vi "Main.vi"() -> ()   [LabVIEW 2018]
doc: "The myRIO Project template acquires acceleration data from the onboard accelerometer and displays the changes of acceleration values in a waveform chart."
uses:
  <vilib>/myRIO/Instrument Drivers/Onboard IO/SPI/typedefs/SPI User Configuration.ctl
  <vilib>/myRIO/Common/Instrument Driver Framework/myRIO v1.0/SPI/typedefs/SPI Clock Phase.ctl
  <vilib>/myRIO/Common/Instrument Driver Framework/myRIO v1.0/SPI/typedefs/SPI Clock Polarity.ctl
  <vilib>/myRIO/Common/Instrument Driver Framework/myRIO v1.0/SPI/typedefs/SPI Data Direction.ctl
  <vilib>/myRIO/Common/Instrument Driver Framework/myRIO v1.0/SPI/typedefs/SPI Frame Length.ctl
  <vilib>/myRIO/Common/Instrument Driver Framework/myRIO v1.0/UART/vis/myRIO v1.0 Close UART.vi
  <vilib>/myRIO/Common/Instrument Driver Framework/Utilities/vis/FPGA Ref Manager.vi
  <vilib>/myRIO/Common/Instrument Driver Framework/myRIO v1.0/myRIO v1.0 Reset FPGA.vi
  <vilib>/myRIO/Common/Instrument Driver Framework/myRIO v1.0/IRQ/vis/myRIO v1.0 IRQ Info FGV.vi
  <vilib>/myRIO/Common/Instrument Driver Framework/myRIO v1.0/IRQ/vis/myRIO v1.0 Timer IRQ Info FGV.vi
  <vilib>/myRIO/Common/Instrument Driver Framework/myRIO v1.0/IRQ/vis/myRIO v1.0 ISR Agent.vi
  <vilib>/myRIO/Instrument Drivers/Utilities/Utilities.lvlib
  <vilib>/myRIO/Instrument Drivers/Onboard IO/SPI/SPI.lvlib
panel:
  out "Data Channel 0":u16[](array[numeric])
  out "Ch0 Distance (cm)":dbl
  out "Ch1 Distance (cm)":dbl
  out "Ch2 Distance (cm)":dbl
  out "Readings good?":bool[](array[boolean])
  out "error out":errorcluster
  in  "Stop":bool
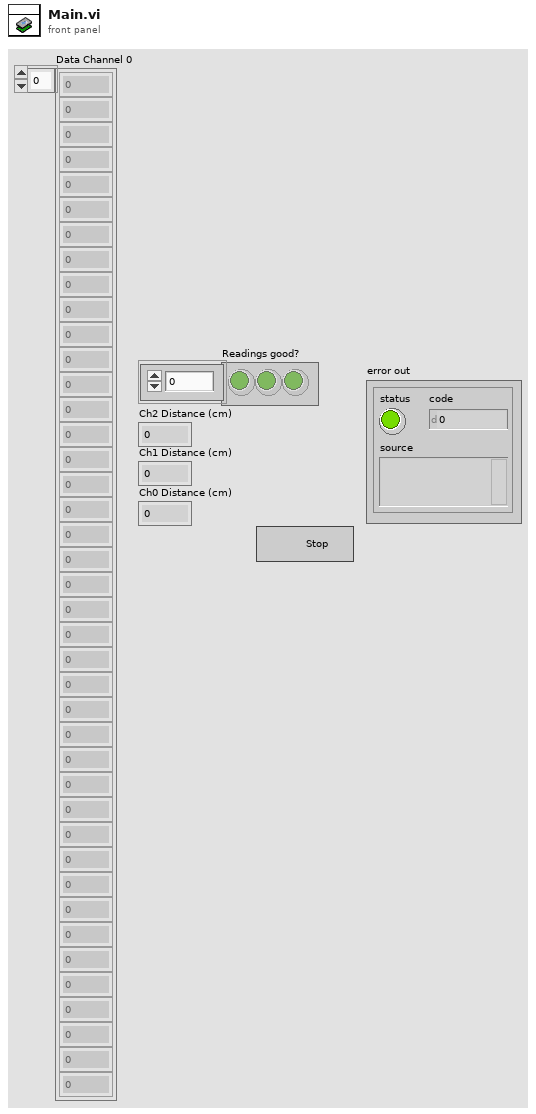
[diagram p1: front panel]
types:
  T1 = typedef "SPI.lvlib/SPI User Configuration.ctl" = cluster{"Frequency [Hz]":dbl, "Clock Phase":T2, "Clock Polarity":T3, "Data Direction":T4, "Frame Length":T5}
  T2 = typedef "SPI Clock Phase.ctl" = enum8{"Leading", "Trailing"}
  T3 = typedef "SPI Clock Polarity.ctl" = enum8{"Low", "High"}
  T4 = typedef "SPI Data Direction.ctl" = enum8{"Most significant bit first", "Least significant bit first"}
  T5 = typedef "SPI Frame Length.ctl" = u8
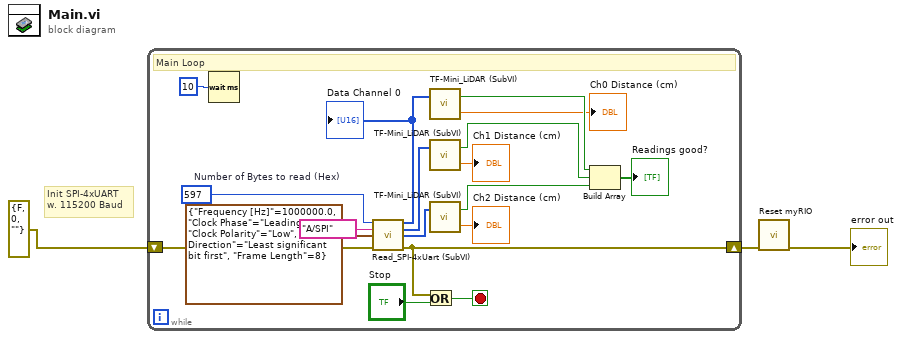
[diagram p0: block diagram]
diagram:
  # "Init SPI-4xUART \nw. 115200 Baud"
  n1 = while {
    shift-right: [w17] -> w3
    shift-left: errorcluster {"status"=FALSE, "code"=0, "source"=""} ("error in (no error)") -> [w18]
    stop <- w20 stop-if-true
    w5 = u32 597  # Number of Bytes to read (Hex)
    # "Main Loop"
    n2 = Wait (ms)(milliseconds to wait=u32 10) -> ()  [unwired: 1 out]
    n3 = call "Read_SPI-4xUart (SubVI).vi"("Number of Bytes to read (Hex)"=w5, "Channel Name"=tag "A/SPI", "SPI User Configuration"=T1 {"Frequency [Hz]"=1000000.0, "Clock Phase"=enum."Leading", "Clock Polarity"=enum."Low", "Data Direction"=enum."Least significant bit first", "Frame Length"=8}, "error in (no error)"=w18) -> ("Data Channel 0"=w15:u16[], "Data Channel 1"=w14:u16[], "Data Channel 2"=w13:u16[], "error out"=w17:errorcluster)  [unwired: 7 in, 1 out]
    "Data Channel 0" <- w15
    n4 = Or(x=w17, y="Stop") -> (x .or. y?=w20:bool)
    n5 = call "TF-Mini_LiDAR (SubVI).vi"("UART Data"=w15) -> ("Distance (cm)"=→"Ch0 Distance (cm)":dbl, "Reading good?"=w12:bool)  [unwired: 1 in]
    n6 = call "TF-Mini_LiDAR (SubVI).vi"("UART Data"=w14) -> ("Distance (cm)"=→"Ch1 Distance (cm)":dbl, "Reading good?"=w11:bool)  [unwired: 1 in]
    n7 = call "TF-Mini_LiDAR (SubVI).vi"("UART Data"=w13) -> ("Distance (cm)"=→"Ch2 Distance (cm)":dbl, "Reading good?"=w10:bool)  [unwired: 1 in]
    n8 = Build Array(w12, w11, w10) -> (→"Readings good?":bool[])
  }
  n9 = call <vilib>:"Reset myRIO.vi"("error in (no error)"=w3) -> ("error out"=→"error out":errorcluster)  [unwired: 10 in]
